vi "HFRR ADV v025 new software.vi"() -> ()   [LabVIEW 2025] (continued)
            n3375 = local read "S 49"() -> (w4577:string)
            n3376 = local read "S 52"() -> (w4574:string)
            n3377 = local read "as"() -> (w4559:string)
            n3378 = local read "bs"() -> (w4560:string)
            n3379 = local read "S 56"() -> (w4573:string)
            n3380 = local read "S 57"() -> (w4572:string)
            n3381 = local read "S 58"() -> (w4571:string)
            n3382 = local read "S 59"() -> (w4570:string)
            n3383 = property on="OPEN" class="Bool (strict)"("Boolean Text.Text"=w4574) -> ()  [unwired: 2 in, 2 out]
            n3384 = property on="OPEN 1" class="Bool (strict)"("Boolean Text.Text"=w4578) -> ()  [unwired: 2 in, 2 out]
            n3385 = property on="OPEN 2" class="Bool (strict)"("Boolean Text.Text"=w4577) -> ()  [unwired: 2 in, 2 out]
            n3386 = property on="OPEN 3" class="Bool (strict)"("Boolean Text.Text"=w4576) -> ()  [unwired: 2 in, 2 out]
            n3387 = property on="OPEN 4" class="Bool (strict)"("Boolean Text.Text"=w4575) -> ()  [unwired: 2 in, 2 out]
            n3388 = Concatenate Strings(w4560, "\r", w4559) -> ()  [unwired: 1 out]
            n3389 = local read "S 102"() -> (w4533:string)
            n3390 = property on="КОФ1" class="DigNum (strict)"("Caption.Text"=w4573) -> ()  [unwired: 2 in, 2 out]
            n3391 = local read "S 98"() -> (w4537:string)
            n3392 = local read "S 99"() -> (w4536:string)
            n3393 = local read "S 100"() -> (w4535:string)
            n3394 = local read "S 101"() -> (w4534:string)
            n3395 = property on="КОФ2" class="DigNum (strict)"("Caption.Text"=w4572) -> ()  [unwired: 2 in, 2 out]
            n3396 = property on="КОФ3" class="DigNum (strict)"("Caption.Text"=w4571) -> ()  [unwired: 2 in, 2 out]
            n3397 = property on="КОФ4" class="DigNum (strict)"("Caption.Text"=w4570) -> ()  [unwired: 2 in, 2 out]
            n3398 = local read "bs"() -> (w4558:string)
            n3399 = local read "as"() -> (w4557:string)
            n3400 = local read "S 60"() -> (w4569:string)
            n3401 = local read "S 54"() -> (w4579:string)
            n3402 = Concatenate Strings(w4558, "\r", w4557) -> ()  [unwired: 1 out]
            n3403 = Concatenate Strings(w4579, w4569) -> ()  [unwired: 1 out]
            n3404 = local read "S 77"() -> (→"String 43":string)
            n3405 = local read "S 76"() -> (w4552:string)
            n3406 = local read "S 78"() -> (w4551:string)
            n3407 = local read "S 71"() -> (w4563:string)
            n3408 = local read "S 66"() -> (w4568:string)
            n3409 = local read "S 67"() -> (w4567:string)
            n3410 = local read "S 68"() -> (w4566:string)
            n3411 = local read "S 69"() -> (w4565:string)
            n3412 = local read "S 70"() -> (w4564:string)
            n3413 = property on="AIR TEMP" class="DigNum (strict)"("Caption.Text"=w4551) -> ()  [unwired: 2 in, 2 out]
            n3414 = property on="Set Strk" class="DigNum (strict)"("Caption.Text"=w4552) -> ()  [unwired: 2 in, 2 out]
            n3415 = property on="SPEED OUT:" class="DigNum (strict)"("Caption.Text"=w4566) -> ()  [unwired: 2 in, 2 out]
            n3416 = property on="EDIT" class="Bool (strict)"("Boolean Text.Text"=w4563) -> ()  [unwired: 2 in, 2 out]
            n3417 = local read "S 79"() -> (w4550:string)
          }
          frame #2 {
          }
        }
        n3418 = local write "Lan flag"(10.0 ("Lan flag")) -> ()
      }
      frame Enabled {
      }
    }
    n3419 = Wait (ms)(milliseconds to wait=u32 2000) -> ()  [unwired: 1 out]
    n3420 = local read "Quit"() -> (w4353:bool)
  }
  n3421 = while {
    shift-right: [w4585] -> _
    shift-left: _ -> [w4586]
    shift-right: [w4583] -> _
    shift-left: T16 {"Read Heave and Surge"="", "Bytes at Heave Port"=0.0, "Heave and Surge COM Port:"="COM9", "Com Port 2"="COM7", "Residual Due"="", "Heave COM Status 2"=TRUE, "Heave COM Status"=TRUE, "Port 2"=TRUE, "Sway PPR"=6400.0, "Surge PPR"=6400.0, "Heave PPR"=6400.0, "Sway Pitch"=2.0, "Surge Pitch"=3.0, "Heave Pitch"=4.0, "Sway Pulses/mm"=320.0, "Surge Pulses/mm"=1600.0, "Heave Pulses/mm"=1600.0, "inner loop"=0.0, "Read Heave and Surge 2"="", "String 36"="", "Write S"=FALSE, "WriteCC1"=[""], "Heave COM Loop"=0, "LastCom"="", "EXIT"=FALSE, "Error Heave"={"status"=TRUE, "code"=-1073807343, "source"=""}} -> [w4582]
    shift-right: [w4580] -> _
    shift-left: enum16{"init", "MAIN", "Panel Close"}."init" -> [w4581]
    stop <- w4584 stop-if-true
    # "HUMIDITY LOOP LOGIC"
    n3422 = case shown="\"MAIN\"" w4581 {
      tunnel: w4586 -> [w4600 w4617 w4674 w4676]
      tunnel: [w4595 w4622 w4674 w4676] -> w4585
      tunnel: [_ _ TRUE _] -> w4584
      tunnel: [w4592 w4620 w4672 w4675] -> w4583
      tunnel: w4582 -> [w4597 w4616 w4672 w4675]
      tunnel: [enum16{"init", "MAIN", "Panel Close"}."MAIN" w4611 _ _] -> w4580
      frame "init" {
        n3423 = local read "Com Port 1"() -> (w4589:refnum<visa-resource-name>)
        n3424 = Bundle By Name(cluster=w4597, "Heave and Surge COM Port:"=w4589) -> (w4596:T16)
        n3425 = call "Instrument fgv uno.vi"("Enum"=T29."INIT", "error in (no error) 2"=w4600, "INPUT"=w4596) -> ("error"=w4598:errorcluster, "output"=w4594:T16)  [unwired: 6 in, 1 out]
        n3426 = case shown="Error" w4598 {
          selector: w4598 -> [w4602 _]
          tunnel: [w4602 w4606] -> w4595
          tunnel: w4594 -> [w4601 w4604]
          tunnel: [w4601 w4603] -> w4593
          frame No Error {
          }
          frame Error {
            n3427 = call "Instrument fgv uno.vi"("Enum"=T29."ERROR INIT", "INPUT"=w4604) -> ("error"=w4607:errorcluster, "output"=w4603:T16)  [unwired: 7 in, 1 out]
            n3428 = call <vilib>:"Clear Errors.vi"("error in (no error)"=w4607) -> ("error out"=w4606:errorcluster)  [unwired: 5 in, 1 out]
          }
        }
        n3429 = local read "LastCom Humidity"() -> (w4588:string)
        n3430 = Unbundle By Name(w4593) -> ("Heave COM Status 2"=→"COM Status":bool, "Error Heave"=→"Error  2":errorcluster)  [unwired: 1 out]
        n3431 = Bundle By Name(cluster=w4593, "LastCom"=w4588) -> (w4592:T16)
      }
      frame "MAIN" {
        n3432 = Unbundle By Name(w4616) -> ("Com Port 2"=w4624:refnum<visa-resource-name>)
        n3433 = local read "Com Port 1"() -> (w4610:refnum<visa-resource-name>)
        n3434 = local write "Com Port 5"(w4624) -> ()
        n3435 = Bundle By Name(cluster=w4616, "Heave and Surge COM Port:"=w4610) -> (w4615:T16)
        n3436 = Equal?(x=w4624, y=w4610) -> (x = y?=w4623:bool)
        n3437 = case shown="True" w4623 {
          tunnel: [w4628 w4645] -> w4622
          tunnel: w4617 -> [w4629 w4651]
          tunnel: w4615 -> [w4627 w4649]
          tunnel: [w4626 w4644] -> w4620
          frame False {
            n3438 = call <vilib>:"Clear Errors.vi"("error in (no error)"=w4629) -> ("error out"=w4625:errorcluster)  [unwired: 5 in, 1 out]
            n3439 = call "Instrument fgv uno.vi"("Enum"=T29."ERROR INIT", "error in (no error) 2"=w4625, "INPUT"=w4627) -> ("error"=w4631:errorcluster, "output"=w4626:T16)  [unwired: 6 in, 1 out]
            n3440 = call <vilib>:"Clear Errors.vi"("error in (no error)"=w4631) -> ("error out"=w4628:errorcluster)  [unwired: 5 in, 1 out]
          }
          frame True {
            n3441 = call "Instrument fgv uno.vi"("Enum"=T29."READ", "error in (no error) 2"=w4651, "INPUT"=w4649) -> ("error"=w4650:errorcluster, "output"=w4642:T16)  [unwired: 6 in, 1 out]
            n3442 = Bundle By Name(cluster=w4642, "String 36"="WRITE HUMIDITY") -> (w4641:T16)
            n3443 = case shown="True" "Write" {
              selector: "Write" -> [_ w4671]
              tunnel: w4650 -> [w4664 w4670]
              tunnel: [w4664 w4669] -> w4639
              tunnel: w4641 -> [w4663 w4666]
              tunnel: [w4663 w4665] -> w4638
              frame False {
              }
              frame True {
                n3444 = Not(x=w4671) -> (.not. x?=w4667:bool)
                n3445 = local write "Write"(w4667) -> ()
                n3446 = call "Instrument fgv uno.vi"("Enum"=T29."MANUAL WRITE", "error in (no error) 2"=w4670, "INPUT"=w4666) -> ("error"=w4669:errorcluster, "output"=w4665:T16)  [unwired: 6 in, 1 out]
              }
            }
            n3447 = Array Size(array="WriteHumidity") -> (size(s)=w4636:i32)
            n3448 = Greater Than 0?(x=w4636) -> (x > 0?=w4635:bool)
            n3449 = call "Instrument fgv uno.vi"("Enum"=T29."WRITE", "error in (no error) 2"=w4639, "WriteCC1"="WriteHumidity", "INPUT"=w4638) -> ("error"=w4647:errorcluster, "WriteCC1 2"=w4637:string[], "output"=w4646:T16)  [unwired: 5 in]
            n3450 = case shown="True" w4635 {
              tunnel: w4637 -> [_ w4653]
              frame False {
              }
              frame True {
                n3451 = local write "WriteHumidity"(w4653) -> ()
              }
            }
            n3452 = case shown="No Error" w4647 {
              selector: w4647 -> [w4654 w4657]
              tunnel: w4646 -> [w4655 w4662]
              tunnel: [w4655 w4661] -> w4644
              tunnel: [w4654 w4659] -> w4645
              frame No Error {
              }
              frame Error {
                n3453 = call <vilib>:"Clear Errors.vi"("error in (no error)"=w4657) -> ("error out"=w4656:errorcluster)  [unwired: 5 in, 1 out]
                n3454 = call "Instrument fgv uno.vi"("Enum"=T29."ERROR INIT", "error in (no error) 2"=w4656, "INPUT"=w4662) -> ("error"=w4660:errorcluster, "output"=w4661:T16)  [unwired: 6 in, 1 out]
                n3455 = call <vilib>:"Clear Errors.vi"("error in (no error)"=w4660) -> ("error out"=w4659:errorcluster)  [unwired: 5 in, 1 out]
              }
            }
            n3456 = Unbundle By Name(w4644) -> ("LastCom"=→"LastCom Humidity":string, "Read Heave and Surge"=→"Read HUMIDITY":string)
          }
        }
        n3457 = Unbundle By Name(w4620) -> ("Heave COM Status 2"=w4621:bool, "Error Heave"=w4618:errorcluster, "Bytes at Heave Port"=→"Bytes at Humidity Port  2":dbl)  [unwired: 1 out]
        n3458 = Unbundle By Name(w4618) -> ("status"=→"Humidity Port":bool)
        n3459 = Not(x=w4621) -> (.not. x?=w4608:bool)
        n3460 = local read "Quit"() -> (w4612:bool)
        n3461 = local write "COM Status"(w4608) -> ()
        n3462 = Select(t=enum16{"init", "MAIN", "Panel Close"}."Panel Close", s=w4612, f=enum16{"init", "MAIN", "Panel Close"}."MAIN") -> (s? t:f=w4611:enum16{"init", "MAIN", "Panel Close"})
      }
      frame "Panel Close" {
      }
      frame Default {
      }
    }
  }
  n3463 = disable-structure shown="Disabled" {
    frame Disabled {
      n3464 = while {
        tunnel: [w4678] -> _
        i -> [w4678]
        stop <- w4677 continue-if-true
        n3465 = Wait (ms)(milliseconds to wait=u32 50) -> ()  [unwired: 1 out]
        n3466 = stacked-sequence {
          frame #0 {
            # "Controls Text color"
            # "Controls BG color"
            n3467 = property on="FILE" class="Str"("Text.Text Colors:Text Color"="SC  Text") -> ()  [unwired: 2 in, 2 out]
            n3468 = property on="Fuel Discription :" class="Str"("Text.Text Colors:Text Color"="SC  Text") -> ()  [unwired: 2 in, 2 out]
            n3469 = property on="tested by" class="Str"("Text.Text Colors:Text Color"="SC  Text") -> ()  [unwired: 2 in, 2 out]
            n3470 = property on="Remarks :" class="Str"("Text.Text Colors:Text Color"="SC  Text") -> ()  [unwired: 2 in, 2 out]
            n3471 = property class="DigNum (strict)"("Numeric Text.Text Colors:BG Color"="NC BG") -> ()  [unwired: 2 in, 2 out]
            n3472 = property class="DigNum (strict)"("Numeric Text.Text Colors:BG Color"="NC BG") -> ()  [unwired: 2 in, 2 out]
            n3473 = property class="DigNum (strict)"("Numeric Text.Text Colors:BG Color"="NC BG") -> ()  [unwired: 2 in, 2 out]
            n3474 = property class="DigNum (strict)"("Numeric Text.Text Colors:BG Color"="NC BG") -> ()  [unwired: 2 in, 2 out]
            n3475 = property class="DigNum (strict)"("Numeric Text.Text Colors:BG Color"="NC BG") -> ()  [unwired: 2 in, 2 out]
            n3476 = property class="DigNum (strict)"("Numeric Text.Text Colors:BG Color"="NC BG") -> ()  [unwired: 2 in, 2 out]
            n3477 = property class="DigNum (strict)"("Numeric Text.Text Colors:BG Color"="NC BG") -> ()  [unwired: 2 in, 2 out]
            n3478 = property class="DigNum (strict)"("Numeric Text.Text Colors:BG Color"="NC BG") -> ()  [unwired: 2 in, 2 out]
            n3479 = property class="DigNum (strict)"("Numeric Text.Text Colors:BG Color"="NC BG") -> ()  [unwired: 2 in, 2 out]
            n3480 = property class="DigNum (strict)"("Numeric Text.Text Colors:BG Color"="NC BG") -> ()  [unwired: 2 in, 2 out]
            n3481 = property class="DigNum (strict)"("Numeric Text.Text Colors:BG Color"="NC BG") -> ()  [unwired: 2 in, 2 out]
            n3482 = property class="DigNum (strict)"("Numeric Text.Text Colors:BG Color"="NC BG") -> ()  [unwired: 2 in, 2 out]
            n3483 = property on="FILE" class="Str"("Text.Text Colors:BG Color"="SC BG 3") -> ()  [unwired: 2 in, 2 out]
            n3484 = property on="Fuel Discription :" class="Str"("Text.Text Colors:BG Color"="SC BG 3") -> ()  [unwired: 2 in, 2 out]
            n3485 = property on="tested by" class="Str"("Text.Text Colors:BG Color"="SC BG 3") -> ()  [unwired: 2 in, 2 out]
            n3486 = property on="Remarks :" class="Str"("Text.Text Colors:BG Color"="SC BG 3") -> ()  [unwired: 2 in, 2 out]
            n3487 = property class="DigNum (strict)"("Numeric Text.Text Colors:Text Color"="NC Text") -> ()  [unwired: 2 in, 2 out]
            n3488 = property class="DigNum (strict)"("Numeric Text.Text Colors:Text Color"="NC Text") -> ()  [unwired: 2 in, 2 out]
            n3489 = property class="DigNum (strict)"("Numeric Text.Text Colors:Text Color"="NC Text") -> ()  [unwired: 2 in, 2 out]
            n3490 = property class="DigNum (strict)"("Numeric Text.Text Colors:Text Color"="NC Text") -> ()  [unwired: 2 in, 2 out]
            n3491 = property class="DigNum (strict)"("Numeric Text.Text Colors:Text Color"="NC Text") -> ()  [unwired: 2 in, 2 out]
            n3492 = property class="DigNum (strict)"("Numeric Text.Text Colors:Text Color"="NC Text") -> ()  [unwired: 2 in, 2 out]
            n3493 = property class="DigNum (strict)"("Numeric Text.Text Colors:Text Color"="NC Text") -> ()  [unwired: 2 in, 2 out]
            n3494 = property class="DigNum (strict)"("Numeric Text.Text Colors:Text Color"="NC Text") -> ()  [unwired: 2 in, 2 out]
            n3495 = property class="DigNum (strict)"("Numeric Text.Text Colors:Text Color"="NC Text") -> ()  [unwired: 2 in, 2 out]
            n3496 = property class="DigNum (strict)"("Numeric Text.Text Colors:Text Color"="NC Text") -> ()  [unwired: 2 in, 2 out]
            n3497 = property class="DigNum (strict)"("Numeric Text.Text Colors:Text Color"="NC Text") -> ()  [unwired: 2 in, 2 out]
            n3498 = property class="DigNum (strict)"("Numeric Text.Text Colors:Text Color"="NC Text") -> ()  [unwired: 2 in, 2 out]
            n3499 = property class="DigNum (strict)"("Numeric Text.Text Colors:Text Color"="NI Text  2") -> ()  [unwired: 2 in, 2 out]
            n3500 = property class="DigNum (strict)"("Numeric Text.Text Colors:Text Color"="NI Text  2") -> ()  [unwired: 2 in, 2 out]
            n3501 = property class="DigNum (strict)"("Numeric Text.Text Colors:Text Color"="NI Text  2") -> ()  [unwired: 2 in, 2 out]
            n3502 = property class="DigNum (strict)"("Numeric Text.Text Colors:Text Color"="NI Text  2") -> ()  [unwired: 2 in, 2 out]
            n3503 = property class="DigNum (strict)"("Numeric Text.Text Colors:Text Color"="NI Text  2") -> ()  [unwired: 2 in, 2 out]
            n3504 = property class="DigNum (strict)"("Numeric Text.Text Colors:Text Color"="NI Text  2") -> ()  [unwired: 2 in, 2 out]
            n3505 = property class="DigNum (strict)"("Numeric Text.Text Colors:Text Color"="NI Text  2") -> ()  [unwired: 2 in, 2 out]
            n3506 = property class="DigNum (strict)"("Numeric Text.Text Colors:Text Color"="NI Text  2") -> ()  [unwired: 2 in, 2 out]
            n3507 = property class="DigNum (strict)"("Numeric Text.Text Colors:Text Color"="NI Text  2") -> ()  [unwired: 2 in, 2 out]
            n3508 = property class="DigNum (strict)"("Numeric Text.Text Colors:Text Color"="NI Text  2") -> ()  [unwired: 2 in, 2 out]
            n3509 = property class="DigNum (strict)"("Numeric Text.Text Colors:Text Color"="NI Text  2") -> ()  [unwired: 2 in, 2 out]
            n3510 = property class="DigNum (strict)"("Numeric Text.Text Colors:Text Color"="NI Text  2") -> ()  [unwired: 2 in, 2 out]
            n3511 = property class="DigNum (strict)"("Numeric Text.Text Colors:Text Color"="NI Text  2") -> ()  [unwired: 2 in, 2 out]
            n3512 = property class="DigNum (strict)"("Numeric Text.Text Colors:Text Color"="NI Text  2") -> ()  [unwired: 2 in, 2 out]
            n3513 = property class="DigNum (strict)"("Numeric Text.Text Colors:Text Color"="NI Text  2") -> ()  [unwired: 2 in, 2 out]
            n3514 = property on="Coefficient Of Friction" class="XYGraph (strict)"("Plot Area:Colors:FG Color"="GFG  2", "Plot Area:Colors:BG Color"="GBG   2") -> ()  [unwired: 2 in, 2 out]
            n3515 = property on="Humidity ( %RH )" class="XYGraph (strict)"("Plot Area:Colors:FG Color"="GFG  2", "Plot Area:Colors:BG Color"="GBG   2") -> ()  [unwired: 2 in, 2 out]
            n3516 = property on="Air Temperature  ( °C )" class="XYGraph (strict)"("Plot Area:Colors:FG Color"="GFG  2", "Plot Area:Colors:BG Color"="GBG   2") -> ()  [unwired: 2 in, 2 out]
            n3517 = property on="Sample Temperature ( °C )" class="XYGraph (strict)"("Plot Area:Colors:FG Color"="GFG  2", "Plot Area:Colors:BG Color"="GBG   2") -> ()  [unwired: 2 in, 2 out]
            n3518 = property class="DigNum (strict)"("Numeric Text.Text Colors:BG Color"="NI BG 2") -> ()  [unwired: 2 in, 2 out]
            n3519 = property class="DigNum (strict)"("Numeric Text.Text Colors:BG Color"="NI BG 2") -> ()  [unwired: 2 in, 2 out]
            n3520 = property class="DigNum (strict)"("Numeric Text.Text Colors:BG Color"="NI BG 2") -> ()  [unwired: 2 in, 2 out]
            n3521 = property class="DigNum (strict)"("Numeric Text.Text Colors:BG Color"="NI BG 2") -> ()  [unwired: 2 in, 2 out]
            n3522 = property class="DigNum (strict)"("Numeric Text.Text Colors:BG Color"="NI BG 2") -> ()  [unwired: 2 in, 2 out]
            n3523 = property class="DigNum (strict)"("Numeric Text.Text Colors:BG Color"="NI BG 2") -> ()  [unwired: 2 in, 2 out]
            n3524 = property class="DigNum (strict)"("Numeric Text.Text Colors:BG Color"="NI BG 2") -> ()  [unwired: 2 in, 2 out]
            n3525 = property class="DigNum (strict)"("Numeric Text.Text Colors:BG Color"="NI BG 2") -> ()  [unwired: 2 in, 2 out]
            n3526 = property class="DigNum (strict)"("Numeric Text.Text Colors:BG Color"="NI BG 2") -> ()  [unwired: 2 in, 2 out]
            n3527 = property class="DigNum (strict)"("Numeric Text.Text Colors:BG Color"="NI BG 2") -> ()  [unwired: 2 in, 2 out]
            n3528 = property class="DigNum (strict)"("Numeric Text.Text Colors:BG Color"="NI BG 2") -> ()  [unwired: 2 in, 2 out]
            n3529 = property class="DigNum (strict)"("Numeric Text.Text Colors:BG Color"="NI BG 2") -> ()  [unwired: 2 in, 2 out]
            n3530 = property class="DigNum (strict)"("Numeric Text.Text Colors:BG Color"="NI BG 2") -> ()  [unwired: 2 in, 2 out]
            n3531 = property class="DigNum (strict)"("Numeric Text.Text Colors:BG Color"="NI BG 2") -> ()  [unwired: 2 in, 2 out]
            n3532 = property class="DigNum (strict)"("Numeric Text.Text Colors:BG Color"="NI BG 2") -> ()  [unwired: 2 in, 2 out]
            n3533 = property class="Bool"("Colors [4]"="Boolean BC T & BG") -> ()  [unwired: 2 in, 2 out]
            n3534 = property on="Save & Continue" class="Bool (strict)"("Colors [4]"="Boolean BC T & BG") -> ()  [unwired: 2 in, 2 out]
            n3535 = property on="Heater Button" class="Bool (strict)"("Colors [4]"="Boolean BC T & BG") -> ()  [unwired: 2 in, 2 out]
            n3536 = property class="Bool"("Colors [4]"="Boolean BC T & BG") -> ()  [unwired: 2 in, 2 out]
            n3537 = property on="Humidity" class="Bool (strict)"("Colors [4]"="Boolean BC T & BG") -> ()  [unwired: 2 in, 2 out]
            n3538 = property class="Bool (strict)"("Colors [4]"="Boolean BC T & BG") -> ()  [unwired: 2 in, 2 out]
            n3539 = property on="RUN" class="Bool (strict)"("Colors [4]"="Boolean BC T & BG") -> ()  [unwired: 2 in, 2 out]
            n3540 = property on="trip1 8" class="Bool (strict)"("Colors [4]"="Boolean BC T & BG") -> ()  [unwired: 2 in, 2 out]
            n3541 = property class="Bool"("Colors [4]"="Boolean BC T & BG") -> ()  [unwired: 2 in, 2 out]
            n3542 = property class="Bool (strict)"("Colors [4]"="Boolean BC T & BG") -> ()  [unwired: 2 in, 2 out]
            n3543 = property on="OPEN 1" class="Bool (strict)"("Colors [4]"="Boolean BC T & BG 2") -> ()  [unwired: 2 in, 2 out]
            n3544 = property on="OPEN 2" class="Bool (strict)"("Colors [4]"="Boolean BC T & BG 2") -> ()  [unwired: 2 in, 2 out]
            n3545 = property on="OPEN 3" class="Bool (strict)"("Colors [4]"="Boolean BC T & BG 2") -> ()  [unwired: 2 in, 2 out]
            n3546 = property on="OPEN 4" class="Bool (strict)"("Colors [4]"="Boolean BC T & BG 2") -> ()  [unwired: 2 in, 2 out]
            n3547 = property on="OPEN" class="Bool (strict)"("Colors [4]"="Boolean BC T & BG 2") -> ()  [unwired: 2 in, 2 out]
            n3548 = property on="rstv2" class="Bool"("Colors [4]"="Boolean BC T & BG 2") -> ()  [unwired: 2 in, 2 out]
            n3549 = property on="RST CP" class="Bool"("Colors [4]"="Boolean BC T & BG 2") -> ()  [unwired: 2 in, 2 out]
            n3550 = property on="RSTV1 3" class="Bool"("Colors [4]"="Boolean BC T & BG 2") -> ()  [unwired: 2 in, 2 out]
            n3551 = property on="RSTV1 2" class="Bool"("Colors [4]"="Boolean BC T & BG 2") -> ()  [unwired: 2 in, 2 out]
          }
          frame #1 {
          }
        }
        n3552 = local read "Quit"() -> (w4677:bool)
      }
    }
    frame Enabled {
    }
  }
  n3553 = while {
    shift-right: [w4695] -> _
    shift-left: _ -> [w4696]
    shift-right: [w4693] -> _
    shift-left: T16 {"Read Heave and Surge"="", "Bytes at Heave Port"=0.0, "Heave and Surge COM Port:"="COM9", "Com Port 2"="COM7", "Residual Due"="", "Heave COM Status 2"=TRUE, "Heave COM Status"=TRUE, "Port 2"=TRUE, "Sway PPR"=6400.0, "Surge PPR"=6400.0, "Heave PPR"=6400.0, "Sway Pitch"=2.0, "Surge Pitch"=3.0, "Heave Pitch"=4.0, "Sway Pulses/mm"=320.0, "Surge Pulses/mm"=1600.0, "Heave Pulses/mm"=1600.0, "inner loop"=0.0, "Read Heave and Surge 2"="", "String 36"="", "Write S"=FALSE, "WriteCC1"=[""], "Heave COM Loop"=0, "LastCom"="", "EXIT"=FALSE, "Error Heave"={"status"=TRUE, "code"=-1073807343, "source"=""}} -> [w4692]
    shift-right: [w4690] -> _
    shift-left: enum16{"init", "MAIN", "Panel Close"}."init" -> [w4691]
    stop <- w4694 stop-if-true
    # "UNO CODE LOGIC"
    n3554 = case shown="\"MAIN\"" w4691 {
      tunnel: w4696 -> [w4710 w4727 w4785 w4787]
      tunnel: [w4704 w4733 w4785 w4787] -> w4695
      tunnel: [_ _ TRUE _] -> w4694
      tunnel: [w4700 w4731 w4783 w4786] -> w4693
      tunnel: w4692 -> [w4707 w4726 w4783 w4786]
      tunnel: [enum16{"init", "MAIN", "Panel Close"}."MAIN" w4720 _ _] -> w4690
      frame "init" {
        n3555 = Bundle By Name(cluster=w4707, "Heave and Surge COM Port:"="C3 :") -> (w4706:T16)
        n3556 = call "Instrument fgv.vi"("Enum"=T29."INIT", "error in (no error) 2"=w4710, "INPUT"=w4706) -> ("error"=w4708:errorcluster, "output"=w4703:T16)  [unwired: 6 in, 1 out]
        n3557 = case shown="Error" w4708 {
          selector: w4708 -> [w4712 _]
          tunnel: [w4712 w4716] -> w4704
          tunnel: w4703 -> [w4711 w4714]
          tunnel: [w4711 w4713] -> w4701
          frame No Error {
          }
          frame Error {
            n3558 = call "Instrument fgv.vi"("Enum"=T29."ERROR INIT", "INPUT"=w4714) -> ("error"=w4717:errorcluster, "output"=w4713:T16)  [unwired: 7 in, 1 out]
            n3559 = call <vilib>:"Clear Errors.vi"("error in (no error)"=w4717) -> ("error out"=w4716:errorcluster)  [unwired: 5 in, 1 out]
          }
        }
        n3560 = local read "LastCom UNO"() -> (w4697:string)
        n3561 = Unbundle By Name(w4701) -> ("Heave COM Status 2"=→"Instrument Status":bool, "Error Heave"=→"Error":errorcluster)  [unwired: 1 out]
        n3562 = Bundle By Name(cluster=w4701, "LastCom"=w4697) -> (w4700:T16)
      }
      frame "MAIN" {
        n3563 = Unbundle By Name(w4726) -> ("Com Port 2"=w4735:refnum<visa-resource-name>)
        n3564 = local write "Com Port 4"(w4735) -> ()
        n3565 = local read "C3 :"() -> (w4724:refnum<visa-resource-name>)
        n3566 = Bundle By Name(cluster=w4726, "Heave and Surge COM Port:"=w4724) -> (w4725:T16)
        n3567 = Equal?(x=w4735, y=w4724) -> (x = y?=w4734:bool)
        n3568 = case shown="True" w4734 {
          tunnel: [w4739 w4756] -> w4733
          tunnel: w4727 -> [w4740 w4762]
          tunnel: w4725 -> [w4738 w4760]
          tunnel: [w4737 w4755] -> w4731
          frame False {
            n3569 = call <vilib>:"Clear Errors.vi"("error in (no error)"=w4740) -> ("error out"=w4736:errorcluster)  [unwired: 5 in, 1 out]
            n3570 = call "Instrument fgv.vi"("Enum"=T29."ERROR INIT", "error in (no error) 2"=w4736, "INPUT"=w4738) -> ("error"=w4742:errorcluster, "output"=w4737:T16)  [unwired: 6 in, 1 out]
            n3571 = call <vilib>:"Clear Errors.vi"("error in (no error)"=w4742) -> ("error out"=w4739:errorcluster)  [unwired: 5 in, 1 out]
          }
          frame True {
            n3572 = call "Instrument fgv.vi"("Enum"=T29."READ", "error in (no error) 2"=w4762, "INPUT"=w4760) -> ("error"=w4761:errorcluster, "output"=w4753:T16)  [unwired: 6 in, 1 out]
            n3573 = Bundle By Name(cluster=w4753, "String 36"="WRITE UNO") -> (w4752:T16)
            n3574 = case shown="True" "Write S" {
              selector: "Write S" -> [_ w4782]
              tunnel: w4761 -> [w4775 w4781]
              tunnel: [w4775 w4780] -> w4750
              tunnel: w4752 -> [w4774 w4777]
              tunnel: [w4774 w4776] -> w4749
              frame False {
              }
              frame True {
                n3575 = Not(x=w4782) -> (.not. x?=w4778:bool)
                n3576 = local write "Write S"(w4778) -> ()
                n3577 = call "Instrument fgv.vi"("Enum"=T29."MANUAL WRITE", "error in (no error) 2"=w4781, "INPUT"=w4777) -> ("error"=w4780:errorcluster, "output"=w4776:T16)  [unwired: 6 in, 1 out]
              }
            }
            n3578 = Array Size(array="Write UNO") -> (size(s)=w4747:i32)
            n3579 = Greater Than 0?(x=w4747) -> (x > 0?=w4746:bool)
            n3580 = call "Instrument fgv.vi"("Enum"=T29."WRITE", "error in (no error) 2"=w4750, "WriteCC1"="Write UNO", "INPUT"=w4749) -> ("error"=w4758:errorcluster, "WriteCC1 2"=w4748:string[], "output"=w4757:T16)  [unwired: 5 in]
            n3581 = case shown="True" w4746 {
              tunnel: w4748 -> [_ w4764]
              frame False {
              }
              frame True {
                n3582 = local write "Write UNO"(w4764) -> ()
              }
            }
            n3583 = case shown="Error" w4758 {
              selector: w4758 -> [w4765 w4768]
              tunnel: w4757 -> [w4766 w4773]
              tunnel: [w4766 w4772] -> w4755
              tunnel: [w4765 w4770] -> w4756
              frame No Error {
              }
              frame Error {
                n3584 = call <vilib>:"Clear Errors.vi"("error in (no error)"=w4768) -> ("error out"=w4767:errorcluster)  [unwired: 5 in, 1 out]
                n3585 = call "Instrument fgv.vi"("Enum"=T29."ERROR INIT", "error in (no error) 2"=w4767, "INPUT"=w4773) -> ("error"=w4771:errorcluster, "output"=w4772:T16)  [unwired: 6 in, 1 out]
                n3586 = call <vilib>:"Clear Errors.vi"("error in (no error)"=w4771) -> ("error out"=w4770:errorcluster)  [unwired: 5 in, 1 out]
              }
            }
            n3587 = Unbundle By Name(w4755) -> ("LastCom"=→"LastCom UNO":string, "Read Heave and Surge"=→"Read UNO":string)
          }
        }
        n3588 = Unbundle By Name(w4731) -> ("Heave COM Status 2"=w4732:bool, "Heave COM Status"=w4719:bool, "Error Heave"=w4729:errorcluster, "Bytes at Heave Port"=→"Bytes at Humidity Port":dbl)
        n3589 = Unbundle By Name(w4729) -> ()  [unwired: 1 out]
        n3590 = Not(x=w4719) -> (.not. x?=w4728:bool)
        n3591 = local write "Error"(w4729) -> ()
        n3592 = Not(x=w4732) -> (.not. x?=w4718:bool)
        n3593 = local write "Instrument Status"(w4728) -> ()
        n3594 = local write "Port 1a"(w4719) -> ()
        n3595 = local read "Quit"() -> (w4721:bool)
        n3596 = local write "COM Status"(w4718) -> ()
        n3597 = Select(t=enum16{"init", "MAIN", "Panel Close"}."Panel Close", s=w4721, f=enum16{"init", "MAIN", "Panel Close"}."MAIN") -> (s? t:f=w4720:enum16{"init", "MAIN", "Panel Close"})
      }
      frame "Panel Close" {
      }
      frame Default {
      }
    }
  }
  n3598 = while {
    stop <- w4813 stop-if-true
    n3599 = local read "Read HUMIDITY"() -> (w4788:string)
    n3600 = call <vilib>:"High Resolution Polling Wait.vi"("seconds to wait"=0.05) -> ()  [unwired: 10 in, 1 out]
    n3601 = Spreadsheet String To Array(delimiter (Tab)=",", format string="", spreadsheet string=w4788, array type (2D Dbl)=string[] []) -> (array=w4808:string[])
    n3602 = for {
      tunnel: w4808 -> [w4818] mode=indexing
      tunnel: string[] ["STATE;", "SET;", "RH;", "T;", "AMB_RH;", "AMB_T;", "PUMP;", "FAN_IN;", "FAN_OUT;", "DEHUM;", "CURRENT;", "STALL;"] -> [w4817] mode=indexing
      tunnel: [w4816] -> w4807 mode=indexing
      n3603 = Match Pattern(string=w4818, regular expression=w4817) -> (after substring=w4816:string)  [unwired: 1 in, 3 out]
    }
    n3604 = Index Array(array=w4807) -> (element #1=→"STATE :":string, element #2=→"SET :":string, element #3=w4796:string, element #4=→"T :":string, element #5=w4794:string, element #6=→"AMB_T :":string, element #7=→"PUMP :":string, element #8=→"FAN_IN :":string, element #9=→"FAN_OUT :":string, element #10=→"DEHUM :":string, element #11=→"CURRENT :":string, element #12=→"STALL :":string)  [unwired: 12 in]
    "RH :" <- w4796
    "AMB_RH :" <- w4794
    n3605 = Fract/Exp String To Number(string=w4796) -> (number=w4789:dbl)  [unwired: 3 in, 1 out]
    n3606 = Fract/Exp String To Number(string=w4794) -> (number=w4793:dbl)  [unwired: 3 in, 1 out]
    n3607 = local write "Ambient Humidity :"(w4793) -> ()
    n3608 = Equal?(x=w4789, y=0.0) -> (x = y?=w4791:bool)
    n3609 = case shown="True" w4791 {
      tunnel: [w4814 w4815] -> w4790
      tunnel: w4789 -> [w4814 _]
      frame False {
        (unwired) 0.0
        "Humidity temp" <- w4814
      }
      frame True {
        n3610 = local read "Humidity temp"() -> (w4815:dbl)
      }
    }
    "RH Numeric:" <- w4790
    n3611 = local read "Quit"() -> (w4813:bool)
  }
  n3612 = disable-structure shown="Disabled" {
    frame Disabled {
      n3613 = while {
        tunnel: [w5052] -> _
        i -> [w5052]
        stop <- w5049 stop-if-true
        n3614 = local read "powstat"() -> (w5050:bool)
        n3615 = case shown="True" w5050 {
          frame False {
          }
          frame True {
            n3616 = local read "RUN"() -> (w5053:bool)
            n3617 = case shown="True" w5053 {
              frame False {
                w5083 = 65.0 ("y")
                n3618 = local read "Set Hz"() -> (w5111:dbl)
                n3619 = local read "NORMAL LOAD"() -> (w5112:dbl)
                n3620 = Multiply(x=w5111, y=60.0) -> (x*y=w5118:dbl)
                n3621 = Multiply(x=1.2 ("y"), y=0.949) -> (x*y=w5087:dbl)
                n3622 = Multiply(x=1.2 ("y"), y=0.8166) -> (x*y=w5091:dbl)
                n3623 = Multiply(x=1.2 ("y"), y=0.851) -> (x*y=w5086:dbl)
                n3624 = local read "FF 2"() -> (w5110:dbl)
                n3625 = Absolute Value(x=w5118) -> (abs(x)=w5116:dbl)
                n3626 = case shown="13.." w5110 {
                  tunnel: [1 2 3] -> w5108
                  frame 0..10, Default {
                    # "Normal"
                  }
                  frame 11, 12 {
                  }
                  frame 13.. {
                  }
                }
                "FF STATE" <- w5108
                n3627 = local read "TEMP"() -> (w5071:dbl)
                n3628 = local read item#-1() -> (w5085)
                n3629 = Less?(x=w5085, y=w5091) -> (x < y?=w5088:bool)
                n3630 = In Range and Coerce(upper limit=w5087, x=w5085, lower limit=w5086) -> (In Range?=w5089:bool)  [unwired: 1 out]
                n3631 = case shown="3601.." w5116 {
                  tunnel: [1 2 3] -> w5114
                  frame 0..3000, Default {
                    # "Normal"
                  }
                  frame 3001..3600 {
                  }
                  frame 3601.. {
                  }
                }
                n3632 = case shown="11.." w5112 {
                  tunnel: [1 3] -> w5113
                  frame 1..10, Default {
                  }
                  frame 11.. {
                  }
                }
                "NL STATE" <- w5113
                n3633 = Multiply(x=1.2 ("y"), y=0.95) -> (x*y=w5101:dbl)
                n3634 = Multiply(x=w5083, y=0.954) -> (x*y=w5075:dbl)
                n3635 = Or(x=w5088, y=w5089) -> (x .or. y?=w5090:bool)
                n3636 = Greater Or Equal?(x=w5085, y=w5101) -> (x >= y?=w5098:bool)
                n3637 = Multiply(x=w5083, y=0.99) -> (x*y=w5072:dbl)
                n3638 = Greater Or Equal?(x=w5071, y=w5072) -> (x >= y?=w5077:bool)
                n3639 = Greater Or Equal?(x=w5071, y=w5075) -> (x >= y?=w5074:bool)
                n3640 = case shown="0, 1, Default" w5085 {
                  tunnel: [1 3] -> w5102
                  frame 0, 1, Default {
                  }
                  frame 2.. {
                  }
                }
                n3641 = case shown="True" w5098 {
                  tunnel: [1 3] -> w5103
                  frame False {
                  }
                  frame True {
                  }
                }
                n3642 = case shown="True" w5090 {
                  tunnel: [1 2] -> w5104
                  frame False {
                  }
                  frame True {
                  }
                }
                n3643 = case shown="..0" w5071 {
                  tunnel: [2 3 3 1] -> w5078
                  frame 61, 62 {
                  }
                  frame 63.. {
                  }
                  frame ..0 {
                  }
                  frame 10..60, Default {
                  }
                }
                n3644 = case shown="True" w5077 {
                  tunnel: [1 3] -> w5079
                  frame False {
                  }
                  frame True {
                  }
                }
                n3645 = Number To Decimal String(number=w5114) -> (decimal integer string=w5115:string)  [unwired: 1 in]
                n3646 = case shown="True" w5074 {
                  tunnel: [1 2] -> w5080
                  frame False {
                  }
                  frame True {
                  }
                }
                n3647 = Number To Decimal String(number=1) -> (decimal integer string=→"Air temp":string)  [unwired: 1 in]
                n3648 = Number To Decimal String(number=w5108) -> (decimal integer string=→"ff_st":string)  [unwired: 1 in]
                n3649 = local write "sp_st"(w5115) -> ()
                n3650 = Number To Decimal String(number=w5113) -> (decimal integer string=→"nl_st":string)  [unwired: 1 in]
                n3651 = Build Array(w5078, w5079, w5080) -> (w5081:i32[])
                n3652 = Build Array(w5102, w5103, w5104) -> (w5105:i32[])
                n3653 = Array Max & Min(array=w5081) -> (max value=w5082:i32)  [unwired: 3 out]
                n3654 = Array Max & Min(array=w5105) -> (max value=w5106:i32)  [unwired: 3 out]
                n3655 = Number To Decimal String(number=w5082) -> (decimal integer string=w5070:string)  [unwired: 1 in]
                n3656 = Number To Decimal String(number=w5106) -> (decimal integer string=→"Stroke Ln 2":string)  [unwired: 1 in]
                n3657 = local write "temp_st"(w5070) -> ()
              }
              frame True {
                w5168 = 65.0 ("y")
                # "Healthy -1\nWarning -2\nError -3"
                n3658 = local read "TEMP"() -> (w5179:dbl)
                n3659 = local read "NORMAL LOAD"() -> (w5183:dbl)
                n3660 = local read "Set Hz"() -> (w5181:dbl)
                n3661 = Multiply(x=1.2 ("y"), y=0.949) -> (x*y=w5163:dbl)
                n3662 = Multiply(x=1.2 ("y"), y=0.8166) -> (x*y=w5159:dbl)
                n3663 = Multiply(x=1.2 ("y"), y=0.851) -> (x*y=w5164:dbl)
                n3664 = Multiply(x=w5168, y=0.954) -> (x*y=w5175:dbl)
                n3665 = Multiply(x=w5168, y=0.99) -> (x*y=w5178:dbl)
                n3666 = Greater Or Equal?(x=w5179, y=w5178) -> (x >= y?=w5173:bool)
                n3667 = Multiply(x=w5181, y=60.0) -> (x*y=w5187:dbl)
                n3668 = Greater Or Equal?(x=w5179, y=w5175) -> (x >= y?=w5176:bool)
                n3669 = local read "FF 2"() -> (w5182:dbl)
                n3670 = local read item#-1() -> (w5165)
                n3671 = Less?(x=w5165, y=w5159) -> (x < y?=w5162:bool)
                n3672 = In Range and Coerce(upper limit=w5163, x=w5165, lower limit=w5164) -> (In Range?=w5161:bool)  [unwired: 1 out]
                n3673 = Absolute Value(x=w5187) -> (abs(x)=w5185:dbl)
                n3674 = case shown="63.." w5179 {
                  tunnel: [2 3 3 1] -> w5172
                  frame 61, 62 {
                  }
                  frame 63.. {
                  }
                  frame ..0 {
                  }
                  frame 10..60, Default {
                  }
                }
                n3675 = case shown="True" w5173 {
                  tunnel: [1 3] -> w5171
                  frame False {
                  }
                  frame True {
                  }
                }
                n3676 = case shown="True" w5176 {
                  tunnel: [1 2] -> w5170
                  frame False {
                  }
                  frame True {
                  }
                }
                n3677 = Multiply(x=1.2 ("y"), y=0.95) -> (x*y=w5149:dbl)
                n3678 = case shown="1..10, Default" w5183 {
                  tunnel: [1 3] -> w5190
                  frame 1..10, Default {
                  }
                  frame 11.. {
                  }
                }
                n3679 = case shown="0..10, Default" w5182 {
                  tunnel: [1 2 3] -> w5189
                  frame 0..10, Default {
                  }
                  frame 11, 12 {
                  }
                  frame 13.. {
                  }
                }
                n3680 = case shown="3601.." w5185 {
                  tunnel: [1 2 3] -> w5184
                  frame 0..3000, Default {
                    # "Normal"
                  }
                  frame 3001..3600 {
                  }
                  frame 3601.. {
                  }
                }
                n3681 = Or(x=w5162, y=w5161) -> (x .or. y?=w5160:bool)
                n3682 = Greater Or Equal?(x=w5165, y=w5149) -> (x >= y?=w5152:bool)
                n3683 = case shown="0, 1, Default" w5165 {
                  tunnel: [1 3] -> w5148
                  frame 0, 1, Default {
                  }
                  frame 2.. {
                  }
                }
                n3684 = case shown="True" w5152 {
                  tunnel: [1 3] -> w5147
                  frame False {
                  }
                  frame True {
                  }
                }
                n3685 = case shown="True" w5160 {
                  tunnel: [1 2] -> w5146
                  frame False {
                  }
                  frame True {
                  }
                }
                n3686 = Build Array(w5172, w5171, w5170) -> (w5169:i32[])
                n3687 = Number To Decimal String(number=w5184) -> (decimal integer string=→"sp_st":string)  [unwired: 1 in]
                n3688 = Array Max & Min(array=w5169) -> (max value=w5166:i32)  [unwired: 3 out]
                "TEMP STATE" <- w5166
                n3689 = Number To Decimal String(number=w5190) -> (decimal integer string=w5193:string)  [unwired: 1 in]
                n3690 = Number To Decimal String(number=w5189) -> (decimal integer string=w5191:string)  [unwired: 1 in]
                n3691 = Number To Decimal String(number=w5166) -> (decimal integer string=→"temp_st":string)  [unwired: 1 in]
                n3692 = Build Array(w5148, w5147, w5146) -> (w5145:i32[])
                n3693 = local write "nl_st"(w5193) -> ()
                n3694 = local write "ff_st"(w5191) -> ()
                n3695 = Number To Decimal String(number=1) -> (decimal integer string=w5188:string)  [unwired: 1 in]
                n3696 = Array Max & Min(array=w5145) -> (max value=w5144:i32)  [unwired: 3 out]
                n3697 = local write "Air temp"(w5188) -> ()
                n3698 = Number To Decimal String(number=w5144) -> (decimal integer string=w5143:string)  [unwired: 1 in]
                n3699 = local write "Stroke Ln 2"(w5143) -> ()
              }
            }
            n3700 = local read "Stroke Ln 2"() -> (w5055:string)
            n3701 = local read "nl_st"() -> (w5061:string)
            n3702 = local read "ff_st"() -> (w5058:string)
            n3703 = local read "sp_st"() -> (w5059:string)
            n3704 = local read "temp_st"() -> (w5060:string)
            n3705 = local read "Air temp"() -> (w5054:string)
            n3706 = Replace Array Subset(array="in", new element #1=w5061, index #1=1 ("index"), new element #2=w5058, index #2=2 ("index"), new element #3=w5060, index #3=3 ("index"), new element #4=w5059, index #4=4 ("index"), new element #5=w5055, index #5=5 ("index"), new element #6=w5054, index #6=6 ("index"), new element #7="Sensor State" ("new element/subarray"), index #7=0 ("index")) -> (→"out":string[])
          }
        }
        n3707 = Wait (ms)(milliseconds to wait=u32 10) -> ()  [unwired: 1 out]
        n3708 = local read "Quit"() -> (w5049:bool)
      }
      n3709 = while {
        stop <- w5024 stop-if-true
        n3710 = local read "run replace"() -> (w5026:bool)
        n3711 = Wait (ms)(milliseconds to wait=u32 100) -> ()  [unwired: 1 out]
        n3712 = Equal?(x="FLAG 2", y=0.0) -> (x = y?=w5027:bool)
        n3713 = case shown="True" w5027 {
          frame False {
          }
          frame True {
            n3714 = local write "FLAG 2"(100.0 ("FLAG 2")) -> ()
            n3715 = call <vilib>:"Read Characters From File.vi"("file path (dialog if empty)"=path "C:/LAB-IQ-NXT/WO 2449 TT.sig", "convert eol? (no:F)"=FALSE ("append to file? (new file:F)")) -> ("character string"=w5030:string)  [unwired: 4 in, 3 out]
            n3716 = call <vilib>:"Read Characters From File.vi"("file path (dialog if empty)"=path "C:/LAB-IQ-NXT/WO 2449 TRH.sig", "convert eol? (no:F)"=FALSE ("append to file? (new file:F)")) -> ("character string"=w5031:string)  [unwired: 4 in, 3 out]
            n3717 = Decimal String To Number(string=w5030) -> (number=w5032:i32)  [unwired: 2 in, 1 out]
            n3718 = local write "Total No. of Tests"(w5032) -> ()
            n3719 = Decimal String To Number(string=w5031) -> (number=w5035:i32)  [unwired: 2 in, 1 out]
            n3720 = local write "SEN.RUN HRS"(w5035) -> ()
          }
        }
        n3721 = case shown="True" w5026 {
          frame False {
          }
          frame True {
            n3722 = Equal?(x="FLAG 4", y=0.0) -> (x = y?=w5039:bool)
            n3723 = case shown="False" w5039 {
              frame False {
                n3724 = Get Date/Time In Seconds() -> (seconds since 1Jan1904=w5045:timestamp)
                n3725 = local read "START 3"() -> (w5043:dbl)
                n3726 = To Double Precision Float(number=w5045) -> (double precision float=w5044:dbl)
                n3727 = Subtract(x=w5044, y=w5043) -> (x-y=→"SENSOR TIME":dbl)
              }
              frame True {
                n3728 = Get Date/Time In Seconds() -> (seconds since 1Jan1904=w5047:timestamp)
                n3729 = local write "FLAG 4"(100.0 ("FLAG")) -> ()
                n3730 = To Double Precision Float(number=w5047) -> (double precision float=→"START 3":dbl)
              }
            }
          }
        }
        n3731 = local read "Quit"() -> (w5024:bool)
      }
      n3732 = while {
        shift-right: [w4824] -> _
        shift-left: _ -> [w4825]
        tunnel: [w4820] -> _
        i -> [w4820]
        stop <- w4819 stop-if-true
        n3733 = Wait (ms)(milliseconds to wait=u32 50 ("Refresh Rate (ms)")) -> ()  [unwired: 1 out]
        n3734 = local read "Json End Flg"() -> (w4821:bool)
        n3735 = Not(x="Upld AR 2") -> ()  [unwired: 1 out]
        n3736 = local read "Upld AR 2"() -> (w4822:bool)
        n3737 = call "Elapsed Time9"("Time Target (s)"="Sen.Upload Rate (s)", "Reset"=FALSE, "Auto Reset"=TRUE) -> ("Time has Elapsed"=w4831:bool)  [unwired: 9 in, 7 out]
        n3738 = Or(x=w4831, y=w4821) -> (x .or. y?=w4827:bool)
        n3739 = case shown="True" w4827 {
          frame False {
          }
          frame True {
            w4923 = "\"SensorName\":\"" ("string")
            w4893 = " \"},{"
            w4918 = "\",\"SensorState\":\""
            w4920 = "\",\"SensorModelNumber\":\"" ("string")
            w4919 = "\",\"SensorRuntimeHours\":\"" ("string")
            n3740 = local read "model num"() -> (w4917:string[])
            n3741 = local read "Sensor name"() -> (w4936:string[])
            n3742 = local read "run"() -> (w4907:string[])
            n3743 = local read "SENSOR TIME"() -> (w4863:dbl)
            n3744 = local read "out"() -> (w4856:string[])
            n3745 = local read "Total No. of Tests"() -> (w4861:dbl)
            n3746 = Select(t=60.0, s="Run test 3", f=3600.0) -> (s? t:f=w4871:dbl)
            n3747 = Index Array(array=w4917, index #1=1 ("index")) -> (element #1=w4916:string, element #2=w4915:string, element #3=w4914:string, element #4=w4913:string, element #5=w4912:string, element #6=w4911:string)  [unwired: 5 in]
            n3748 = Index Array(array=w4907, index #1=1 ("index")) -> (element #1=w4906:string, element #2=w4905:string, element #3=w4904:string, element #4=w4903:string, element #5=w4902:string, element #6=w4901:string)  [unwired: 5 in]
            n3749 = Index Array(array=w4936, index #1=1 ("index")) -> (element #1=w4935:string, element #2=w4934:string, element #3=w4933:string, element #4=w4932:string, element #5=w4922:string, element #6=w4921:string)  [unwired: 5 in]
            n3750 = Index Array(array=w4856, index #1=1 ("index")) -> (element #1=w4888:string, element #2=w4887:string, element #3=w4886:string, element #4=w4885:string, element #5=w4884:string, element #6=w4883:string)  [unwired: 5 in]
            n3751 = local read "SEN.RUN HRS"() -> (w4859:dbl)
            n3752 = Divide(x=w4863, y=w4871) -> (x/y=w4870:dbl)
            n3753 = Increment(x=w4870) -> (x+1=w4866:dbl)
            n3754 = Number To Decimal String(number=w4866) -> (decimal integer string=→"run hrs":string)  [unwired: 1 in]
            n3755 = Divide(x=w4859, y=3600.0 ("f")) -> (x/y=w4854:dbl)
            n3756 = Round To Nearest(number=w4854) -> (nearest integer value=w4852:dbl)
            n3757 = Number To Decimal String(number=w4852) -> (decimal integer string=w4853:string)  [unwired: 1 in]
            n3758 = Number To Decimal String(number=w4861) -> (decimal integer string=w4862:string)  [unwired: 1 in]
            n3759 = local read "Model No"() -> (w4867:string)
            n3760 = local read "UUID"() -> (w4962:string)
            n3761 = local read "Serial No"() -> (w4966:string)
            n3762 = local read "Secret Key"() -> (w4967:string)
            n3763 = Concatenate Strings("\",\"MachineSerialNumber\":\"" ("string"), w4966) -> (w4970:string)
            n3764 = Concatenate Strings("\",\"ModelNumber\":\"" ("string"), w4867) -> (w4868:string)
            n3765 = Concatenate Strings("\",\"MachineRuntimeHours\":\"" ("string"), w4853) -> (w4971:string)
            n3766 = Concatenate Strings("\",\"MachineRuntimeCycles\":\"", w4862) -> (w4964:string)
            n3767 = Concatenate Strings(w4920, w4916) -> (w4950:string)
            n3768 = Concatenate Strings(w4919, w4906) -> (w4951:string)
            n3769 = Concatenate Strings(w4918, w4888) -> (w4949:string)
            n3770 = Concatenate Strings(w4970, w4868, w4971, w4964) -> (w4973:string)
            n3771 = Concatenate Strings(w4920, w4915) -> (w4947:string)
            n3772 = Concatenate Strings(w4919, w4905) -> (w4946:string)
            n3773 = Concatenate Strings(w4918, w4887) -> (w4948:string)
            n3774 = Concatenate Strings(w4920, w4914) -> (w4942:string)
            n3775 = Concatenate Strings(w4919, w4904) -> (w4943:string)
            n3776 = Concatenate Strings(w4918, w4886) -> (w4941:string)
            n3777 = Concatenate Strings(w4920, w4913) -> (w4939:string)
            n3778 = Concatenate Strings(w4919, w4903) -> (w4938:string)
            n3779 = Concatenate Strings(w4918, w4885) -> (w4940:string)
            n3780 = Concatenate Strings(w4950, w4951, w4949) -> (w4952:string)
            n3781 = Concatenate Strings(w4920, w4912) -> (w4929:string)
            n3782 = Concatenate Strings(w4919, w4902) -> (w4930:string)
            n3783 = Concatenate Strings(w4920, w4911) -> (w4926:string)
            n3784 = Concatenate Strings(w4919, w4901) -> (w4925:string)
            n3785 = Concatenate Strings(w4918, w4884) -> (w4928:string)
            n3786 = Concatenate Strings(w4918, w4883) -> (w4927:string)
            n3787 = Concatenate Strings("{\"SecretKey\":\"", w4967, w4973, "\",\"UUID\" : \"", w4962, "\",\"SensorInformation\":", "[{" ("string")) -> (w4900:string)
            n3788 = Concatenate Strings(w4947, w4946, w4948) -> (w4945:string)
            n3789 = Concatenate Strings(w4942, w4943, w4941) -> (w4944:string)
            n3790 = Concatenate Strings(w4939, w4938, w4940) -> (w4937:string)
            n3791 = Concatenate Strings(w4929, w4930, w4928) -> (w4931:string)
            n3792 = Concatenate Strings(w4926, w4925, w4927) -> (w4924:string)
            n3793 = Concatenate Strings(w4923, w4935, w4952, w4893) -> (w4899:string)
            n3794 = Concatenate Strings(w4923, w4934, w4945, w4893) -> (w4898:string)
            n3795 = Concatenate Strings(w4923, w4933, w4944, w4893) -> (w4897:string)
            n3796 = Concatenate Strings(w4923, w4932, w4937, w4893) -> (w4896:string)
            n3797 = Concatenate Strings(w4923, w4922, w4931, w4893) -> (w4895:string)
            n3798 = Concatenate Strings(w4923, w4921, w4924, "\"}" ("string")) -> (w4894:string)
            n3799 = Concatenate Strings(w4900, w4899, w4898, w4897, w4896, w4895, w4894, "]}" ("string")) -> (w4891:string)
            n3800 = local read "SEN.RUN HRS"() -> (w4858:dbl)
            n3801 = disable-structure shown="Disabled" {
              frame Disabled {
                n3802 = local read "state"() -> (w4977:string[])
                n3803 = Delete From Array(array=w4977, index=0) -> (array with subset deleted=w4975:string[])  [unwired: 1 in, 1 out]
                n3804 = for {
                  N: 6 -> [_]
                  tunnel: w4975 -> [w4988] mode=indexing
                  tunnel: [w4987] -> w4974 mode=indexing
                  n3805 = Equal?(x=w4988, y="Warning") -> (x = y?=w4984:bool)
                  n3806 = Equal?(x=w4988, y="Healthy") -> (x = y?=w4981:bool)
                  n3807 = Select(t="2" ("y"), s=w4984, f="3" ("y")) -> (s? t:f=w4979:string)
                  n3808 = Select(t="1" ("y"), s=w4981, f=w4979) -> (s? t:f=w4987:string)
                }
                "state1" <- w4974
              }
              frame Enabled {
              }
            }
            n3809 = stacked-sequence {
              tunnel: w4891 -> [w4999 _ _]
              tunnel: [_ _ w5015] -> _
              frame #0 {
                (unwired) FALSE ("convert eol (F)")
                w5001 = enum16{"start", "end", "current"}."start" ("pos mode (0:2)")
                n3810 = local read "Path"() -> (w4995:path)
                n3811 = Path To String(path=w4995) -> (string=w5007:string)
                n3812 = Concatenate Strings(w5007, "\\", "Sensor File Name") -> (w5008:string)
                n3813 = local write "standard output 2"(" ") -> ()
                n3814 = String To Path(string=w5008) -> (path=w4998:path)
                n3815 = call <vilib>:"Open_Create_Replace File.vi"("advisory dialog? (display:T)"=FALSE, "function (open:0)"=T30."create or replace", "file path"=w4998) -> ("error out"=w5011:errorcluster, "refnum"=w5010:refnum<file>)  [unwired: 5 in, 2 out]
                n3816 = Set File Position(refnum=w5010, from (0:start)=w5001, error in=w5011) -> (refnum out=w4991:refnum<file>, error out=w4990:errorcluster)  [unwired: 1 in]
                n3817 = Write to Binary File(file (use dialog)=w4991, data=" ", error in=w4990, 5:FALSE ("prepend array or string size? (T)")) -> (refnum out=w5002:refnum<file>, error out=w5003:errorcluster)  [unwired: 2 in, 1 out]
                n3818 = Set File Position(offset (in bytes) (0)=w5001, refnum=w5002, error in=w5003) -> (refnum out=w4994:refnum<file>, error out=w4993:errorcluster)  [unwired: 1 in]
                n3819 = Write to Binary File(file (use dialog)=w4994, data=w4999, error in=w4993, 5:FALSE ("prepend array or string size? (T)")) -> (error out=w4997:errorcluster)  [unwired: 2 in, 2 out]
                n3820 = flat-sequence {
                  tunnel: w4998 -> [w5013]
                  tunnel: w4997 -> [_]
                  frame #0 {
                    n3821 = call <vilib>:"Read Characters From File.vi"("file path (dialog if empty)"=w5013) -> ("character string"=→"Sensor Health JSON string":string)  [unwired: 5 in, 3 out]
                  }
                }
                "SinglePoint  2" <- w4999
              }
              frame #1 {
              }
              frame #2 {
                (unwired) "\"Stored\": true" ("string")
                n3822 = call <vilib>:"System Exec.vi"("run minimized? (F)"=TRUE, "wait until completion? (T)"=TRUE, "working directory"=path "C:/LAB-IQ-NXT", "command line"="C:\\LAB-IQ-NXT\\JPostH.bat") -> ("standard error"=→"Respose From Server 2":string, "standard output"=w5018:string)  [unwired: 4 in, 2 out]
                "standard output 2" <- w5018
                n3823 = Match Pattern(string=w5018, regular expression="JSONH Check String") -> (match substring=w5016:string, offset past match=w5015:i32)  [unwired: 1 in, 2 out]
                n3824 = Equal?(x=w5016, y="JSONH Check String") -> (x = y?=→"Upload \nConfirmed 2":bool)
              }
            }
            n3825 = Divide(x=w4858, y=3600.0 ("f")) -> (x/y=w4851:dbl)
            n3826 = local read "run time"() -> (w4908:string[])
            n3827 = Round To Nearest(number=w4851) -> (nearest integer value=w4850:dbl)
            n3828 = Number To Decimal String(number=w4850) -> (decimal integer string=w4849:string)  [unwired: 1 in]
            n3829 = Index Array(array="Sensor Information", index (col) #1=0 ("disabled index (col)"), index (col) #2=1 ("index (col)"), index (col) #3=2 ("index (col)"), index (col) #4=3 ("index (col)")) -> (element #1=→"Sensor name":string[], element #2=→"model num":string[], element #3=→"run time":string[], element #4=→"state":string[])  [unwired: 4 in]
            n3830 = Insert Into Array(array=w4908, index=1, new element #1=w4849, new element #2=w4849, new element #3=w4849, new element #4=w4849, new element #5=w4849, new element #6=w4849) -> (w4873:string[])
            "run" <- w4873
            n3831 = local read "out"() -> (w4855:string[])
            n3832 = local read "Sensor Information"() -> (w4875:string[][])
            n3833 = Replace Array Subset(array=w4875, new element #1=w4873, index (col) #1=2 ("disabled index (col)"), new element #2=w4855, index (col) #2=3 ("index (col)")) -> (w4874:string[][])  [unwired: 2 in]
            n3834 = local write "Sensor Information"(w4874) -> ()
          }
        }
        n3835 = case shown="True" w4822 {
          frame False {
          }
          frame True {
            n3836 = Equal?(x="FLAG", y=0.0) -> (x = y?=w4839:bool)
            n3837 = case shown="False" w4839 {
              frame False {
                n3838 = Get Date/Time In Seconds() -> (seconds since 1Jan1904=w4845:timestamp)
                n3839 = local read "START 2"() -> (w4843:dbl)
                n3840 = To Double Precision Float(number=w4845) -> (double precision float=w4844:dbl)
                n3841 = Subtract(x=w4844, y=w4843) -> (x-y=→"SENSOR TIME  2":dbl)
              }
              frame True {
                n3842 = Get Date/Time In Seconds() -> (seconds since 1Jan1904=w4847:timestamp)
                n3843 = To Double Precision Float(number=w4847) -> (double precision float=→"START 2":dbl)
                n3844 = local write "FLAG"(100.0 ("FLAG")) -> ()
              }
            }
          }
        }
        n3845 = disable-structure shown="Disabled" {
          disable-tunnel: w4825 -> [w4834 _]
          disable-tunnel: [w4833 _] -> w4824
          frame Disabled {
            n3846 = local read "Json St Flg"() -> (w4832:bool)
            n3847 = case shown="True" w4832 {
              tunnel: w4834 -> [w4835 w4837]
              tunnel: [w4835 w4836] -> w4833
              frame False {
              }
              frame True {
                n3848 = Increment(x=w4837) -> (x+1=w4836:dbl)
                "T cycle" <- w4836
                n3849 = local write "Json St Flg"(FALSE ("Json St Flg")) -> ()
              }
            }
          }
          frame Enabled {
          }
        }
        n3850 = local read "Quit"() -> (w4819:bool)
      }
    }
    frame Enabled {
    }
  }
  n3851 = stacked-sequence {
    tunnel: [w5217] -> w42
    frame #0 {
      w5217 = FALSE ("Upload \nConfirmed")
      n3852 = local write "Upload \nConfirmed"(w5217) -> ()
      n3853 = local write "St Str"("") -> ()
    }
  }
  n3854 = disable-structure shown="Disabled" {
    disable-tunnel: w42 -> [w5218 _]
    frame Disabled {
      n3855 = case shown="True" {
        selector: _ -> [_ _]
        tunnel: w5218 -> [_ w5219]
        frame False {
        }
        frame True {
          n3856 = while {
            tunnel: [w5225] -> _
            tunnel: w5219 -> [_]
            i -> [w5225]
            stop <- w5220 stop-if-true
            n3857 = local read "Json End Flg"() -> (w5224:bool)
            n3858 = Wait (ms)(milliseconds to wait=u32 20 ("Refresh Rate (ms)")) -> ()  [unwired: 1 out]
            n3859 = local read "refresh flag"() -> (w5221:bool)
            n3860 = local read "RUN"() -> (w5222:bool)
            n3861 = And(x=w5222, y=w5221) -> (x .and. y?=w5223:bool)
            n3862 = Or(x=w5223, y=w5224) -> (x .or. y?=w5226:bool)
            "AR Led" <- w5226
            n3863 = case shown="True" w5226 {
              frame False {
              }
              frame True {
                w5243 = "\",\""
                n3864 = local read "UUID"() -> (w5241:string)
                n3865 = local write "refresh flag"(FALSE ("refresh flag")) -> ()
                n3866 = local read "time"() -> (w5230:dbl)
                n3867 = Multiply(x=w5230, y=60.0) -> (x*y=w5229:dbl)
                n3868 = Concatenate Strings("UUID\" : \"", w5241, "\"}") -> (w5244:string)
                n3869 = Number To Fractional String(number=w5229, width (-)=i16 10, precision (6)=i16 4) -> (F-format string=w5258:string)  [unwired: 1 in]
                n3870 = Concatenate Strings("{", "\"Time\":\"", w5258, w5243) -> (w5253:string)
                n3871 = stacked-sequence {
                  tunnel: w5243 -> [w5306 w5314 w5321 w5329 w5337 w5346 w5353]
                  tunnel: [w5307 _ _ _ _ _ _] -> w5257
                  tunnel: [_ w5315 _ _ _ _ _] -> w5256
                  tunnel: [_ _ w5322 _ _ _ _] -> w5255
                  tunnel: [_ _ _ w5331 _ _ _] -> w5254
                  tunnel: w5244 -> [_ _ _ _ _ _ w5364]
                  tunnel: [_ _ _ _ _ _ w5363] -> w5240
                  tunnel: [_ _ _ _ _ w5343 _] -> w5239
                  tunnel: [_ _ _ _ w5336 _ _] -> w5238
                  frame #0 {
                    n3872 = local read "NORMAL LOAD"() -> (w5305:dbl)
                    n3873 = Number To Fractional String(number=w5305, width (-)=i16 10, precision (6)=i16 4) -> (F-format string=w5308:string)  [unwired: 1 in]
                    n3874 = Concatenate Strings("NormalLoad\":\"", w5308, w5306) -> (w5307:string)
                  }
                  frame #1 {
                    n3875 = local read "Temp"() -> (w5313:dbl)
                    n3876 = Number To Fractional String(number=w5313, width (-)=i16 10, precision (6)=i16 4) -> (F-format string=w5316:string)  [unwired: 1 in]
                    n3877 = Concatenate Strings("Temperature\":\"", w5316, w5314) -> (w5315:string)
                  }
                  frame #2 {
                    n3878 = local read "cof"() -> (w5319:dbl)
                    n3879 = Number To Fractional String(number=w5319, width (-)=i16 10, precision (6)=i16 4) -> (F-format string=w5323:string)  [unwired: 1 in]
                    n3880 = Concatenate Strings("FrictionalForce\":\"", w5323, w5321) -> (w5322:string)
                  }
                  frame #3 {
                    n3881 = local read "Set Hz"() -> (w5327:dbl)
                    n3882 = Multiply(x=w5327, y=60.0) -> (x*y=w5326:dbl)
                    n3883 = Number To Fractional String(number=w5326, width (-)=i16 10, precision (6)=i16 4) -> (F-format string=w5332:string)  [unwired: 1 in]
                    n3884 = Concatenate Strings("Speed\":\"", w5332, w5329) -> (w5331:string)
                  }
                  frame #4 {
